vi "Aplicatie_trigger.vi"() -> ()   [LabVIEW 2020]
uses:
  994e1307-8dd3-4d9d-b32b-35e3dfa9da5e.vi
  <instrlib>/Agilent 34401/Agilent 34401.lvlib
  \\bucgroup.buc.infineon.com\sc/Internship/CV/2023/Tektronix DPO MSO 2000 4000 Series/Tektronix DPO MSO 2000 4000 Series.lvlib
panel:
  out "error out 2":errorcluster
  out "error out 4":errorcluster
  out "VISA Refnum out":refnum<visa-resource-name>
  in  "Press for measurement":bool
  in  "error in (no error)":errorcluster
  in  "stop":bool
  in  "Select index of measurement:":string(combo)
  in  "Select channel":string(combo)
  in  "Select state:":string(combo)
  in  "Select measurement":string(combo)
  in  "Select statistics's state:":string(combo)
  in  "Select type of histogram:":string(combo)
  in  "Select channel for histogram:":string(combo)
  in  "Select second  transition:":string(combo)
  in  "Select first transition:":string(combo)
  in  "Select polarity:":string(combo)
  in  "Select second channel:":string(combo)
  in  "Select first channel:":string(combo)
  in  "Press for Delta[ms]":bool
  out "Delta[ms]":string
  in  "Cursors Waveform":string(combo)
  in  "SELECT STATE":string(combo)
  in  "SELECT CHANNEL FOR STATE":string(combo)
  in  "Position":dbl
  in  "Select Horizontal position's state:":string(combo)
  in  "Horizontal":dbl step=1.6e-07
  in  "Horizontal Scale":string(combo)
  in  "SELECT CHANNEL FOR SCALE":string(combo)
  in  "Vertical Scale":dbl
  in  "Linked":string(combo)
  in  "Press for Settings for the horizontal bar cursors":bool
  out "Settings for horizontal bar cursors":string
  in  "Press for Settings for the vertical bar cursors":bool
  out "Settings for VERTICAL bar cursors":string
  in  "Select the units":string(combo)
  in  "Press for Delta[mV]":bool
  out "Delta[mV]":string
  in  "Horizontal Cursor 2":dbl(slide) step=0.01 scale=-10.0..10.0
  in  "Horizontal Cursor 1":dbl(slide) step=0.01 scale=-10.0..10.0
  in  "Vertical Cursor 2":dbl(slide) scale=-2e-05..2e-05
  in  "Vertical Cursor 1":dbl(slide) step=0.01 scale=-2e-05..2e-05
  in  "Dots Only":string(combo)
  in  "Select Record Length":string(combo)
  in  "Select mode":string(combo)
  in  "Select bandwidth:":string(combo)
  in  "Select termination:":string(combo)
  in  "Select invert:":string(combo)
  in  "Select coupling:":string(combo)
  in  "Select channel:":string(combo)
  in  "VISA resource name":refnum<visa-resource-name>="USB0::0x0699::0x0401::C000915::INSTR"
  out "error out":errorcluster
  in  "Delay 2":dbl
  in  "Trig OUT 2":string(combo)
  in  "Burst state 2":string(combo)
  in  "Trigger Setup 2":string(combo)
  in  "Number of cycles 2":dbl
  in  "Edge Time 2":dbl
  in  "Pulse Width 2":dbl
  in  "HighLevel 2":dbl
  in  "LowLevel 2":dbl
  in  "Amplitude 2":dbl
  in  "Select function":string(combo)
  in  "Period 2":dbl
  in  "Delay":dbl
  in  "Trig OUT":string(combo)
  in  "Burst state":string(combo)
  in  "Trigger Setup":string(combo)
  in  "Number of cycles":dbl
  in  "Edge Time":dbl
  in  "Pulse Width":dbl
  in  "HighLevel":dbl
  in  "LowLevel":dbl
  in  "Amplitude":dbl
  in  "Select function":string(combo)
  in  "Period":dbl
  # "Configure left waveform generator"
  # "Configure right waveform generator"
  # "Trigger Error"
  # "Measure"
  # "Channel Config"
  # "Acquire"
  # "Add measurement:"
  # "Configure Delay:"
  # "Statistics's state:"
  # "Waveform Histograms:"
  # "Cursors"
  # "Vertical  position"
  # "Vertical scale"
  # "Channel Management"
  # "Horizontal scale"
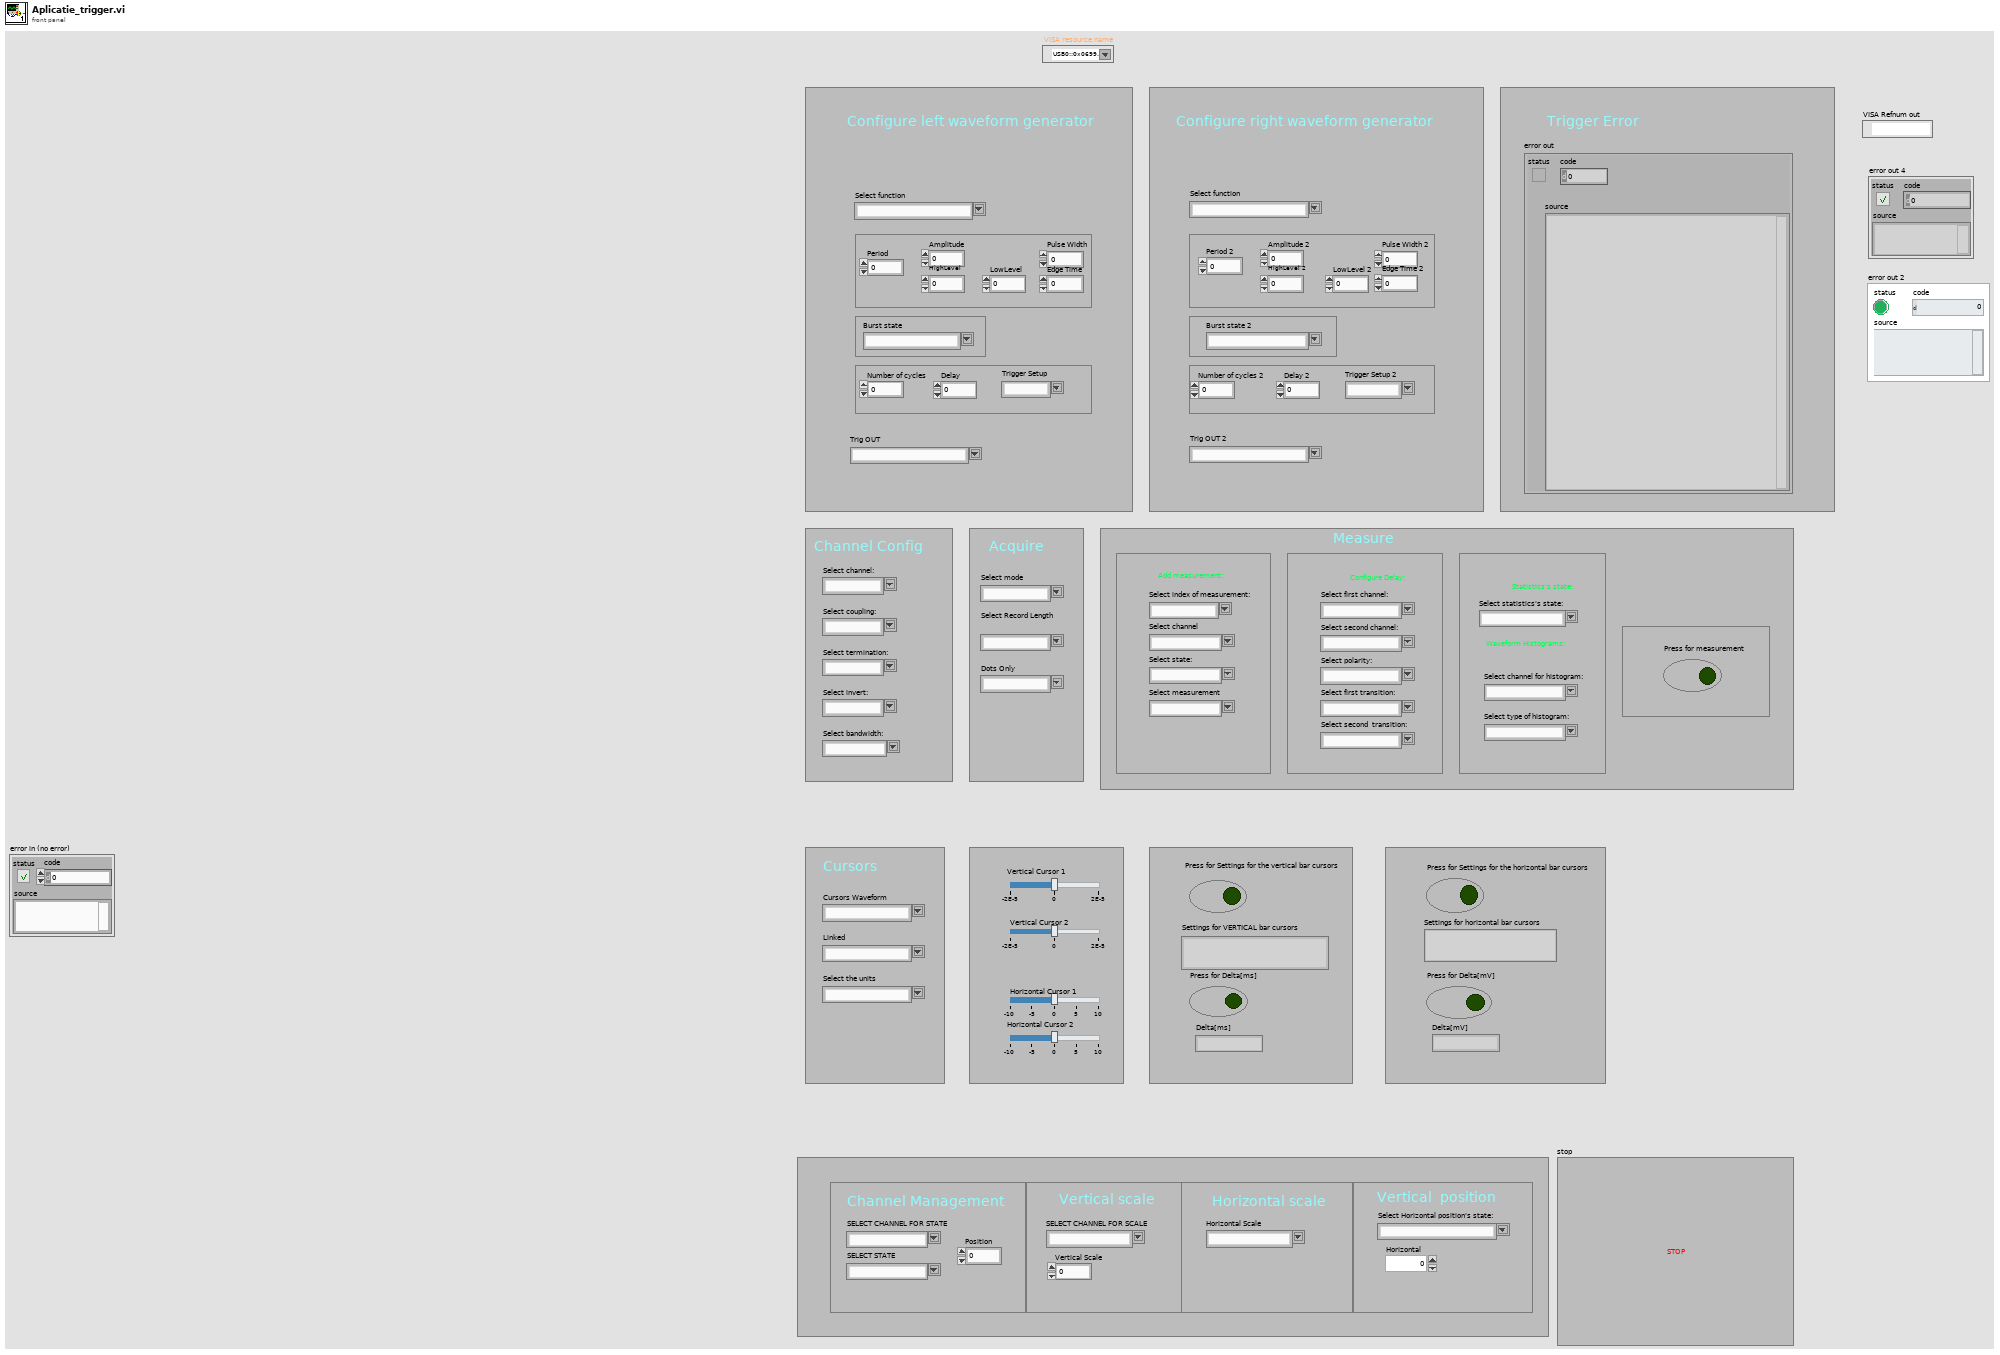
[diagram p1: front panel]
types:
  T1 = enum16{"open", "open or create", "create or replace", "create", "open (read-only)"}
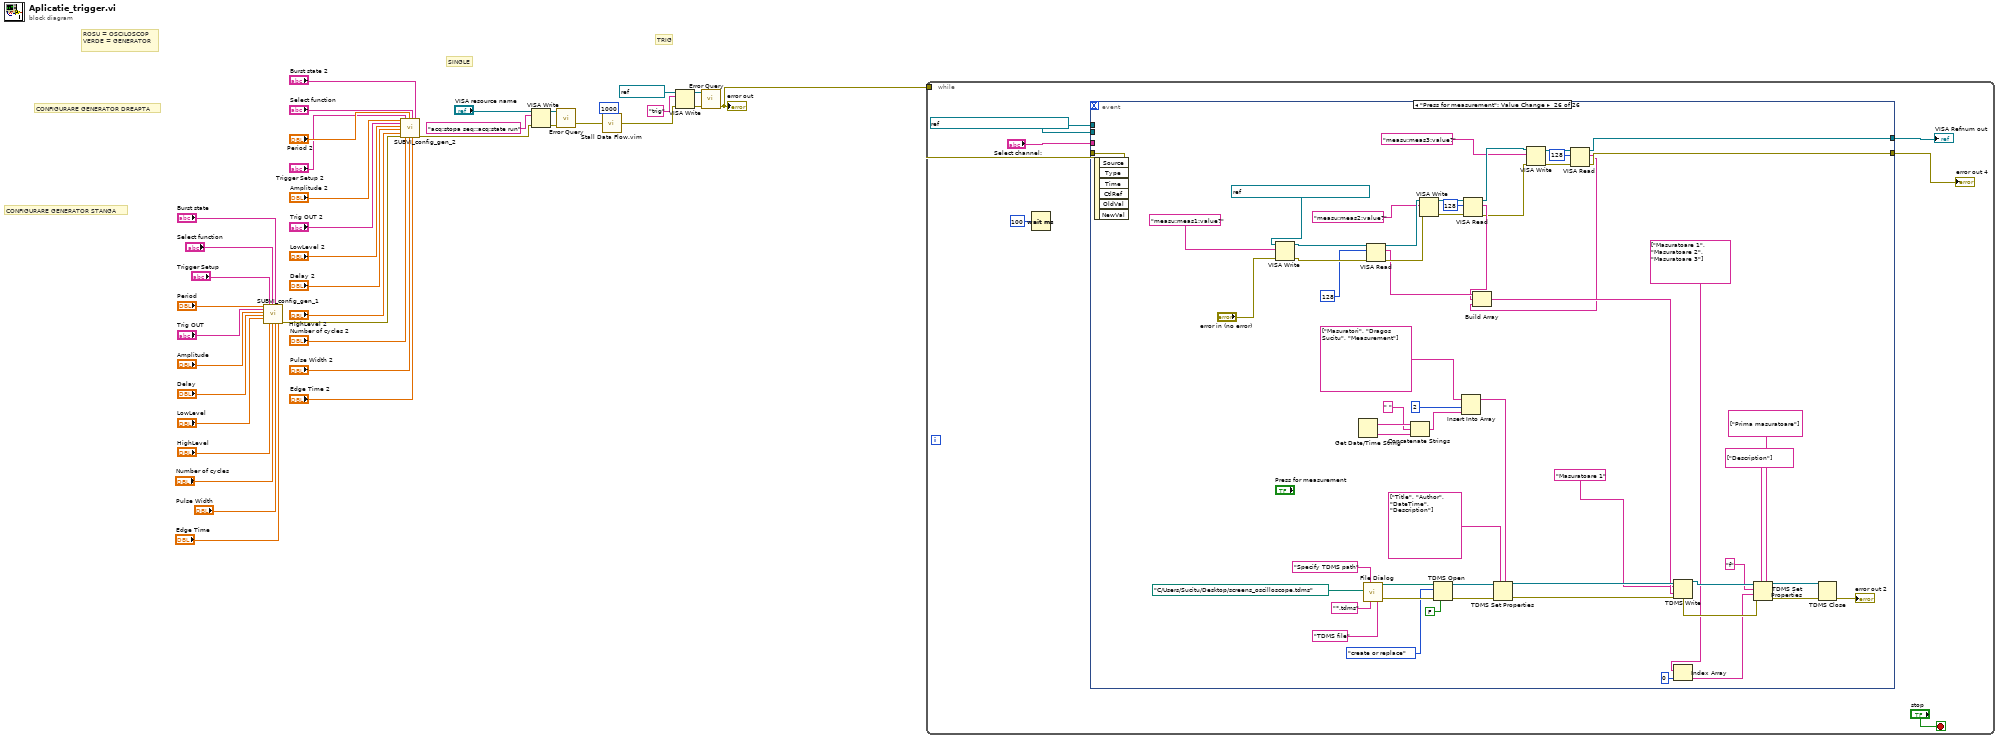
[diagram p0: block diagram]
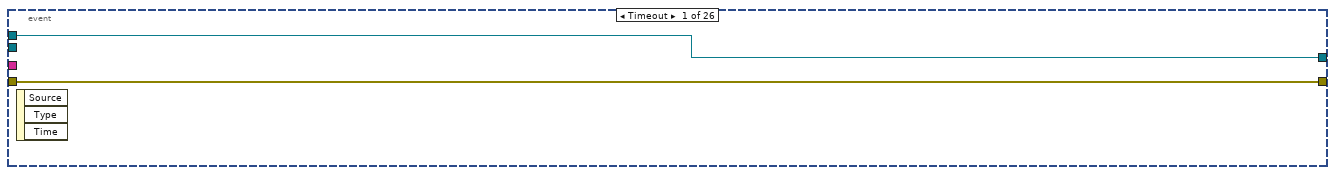
[diagram p2: hidden frame]
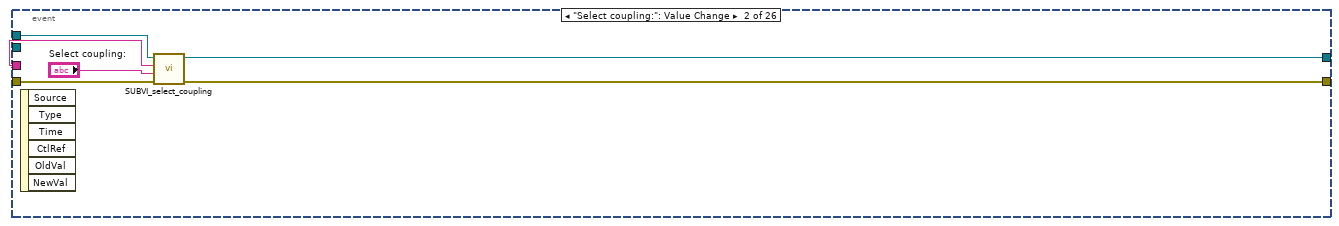
[diagram p3: hidden frame]
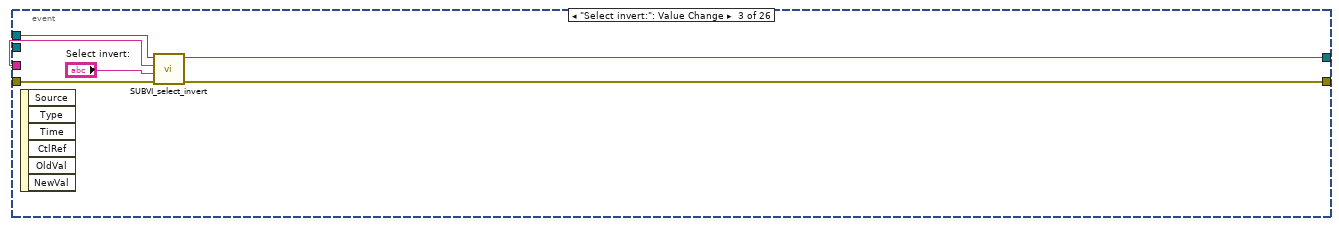
[diagram p4: hidden frame]
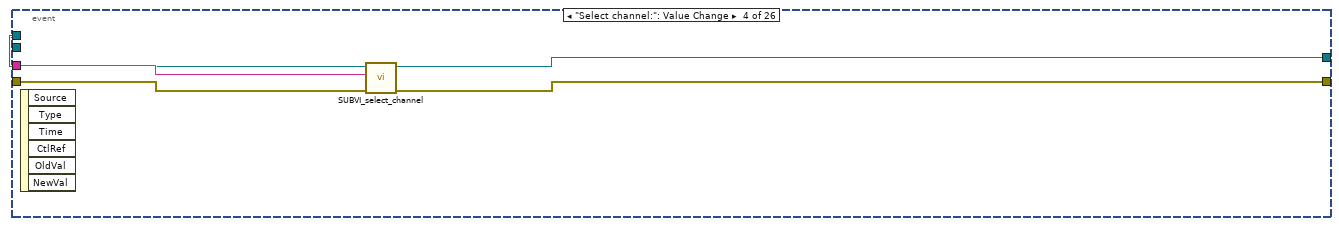
[diagram p5: hidden frame]
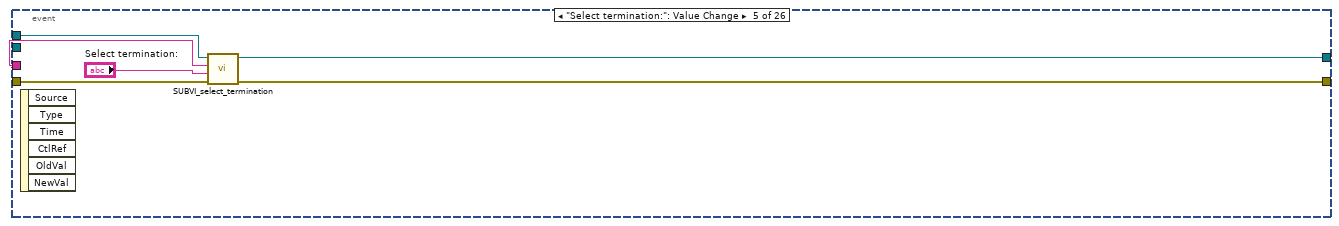
[diagram p6: hidden frame]
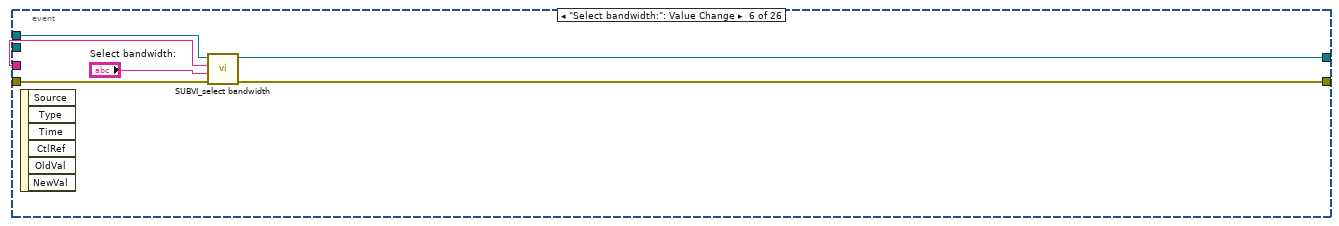
[diagram p7: hidden frame]
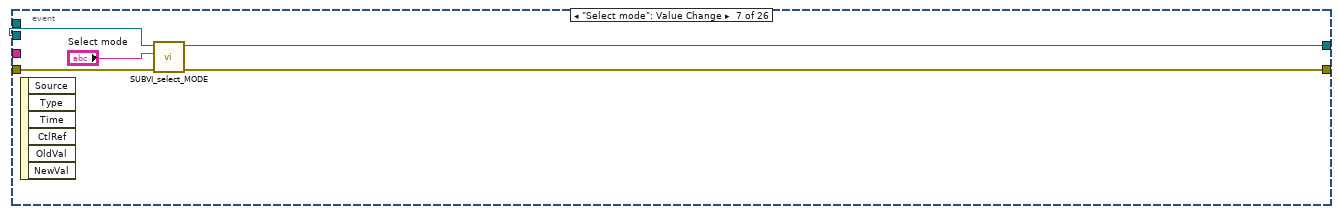
[diagram p8: hidden frame]
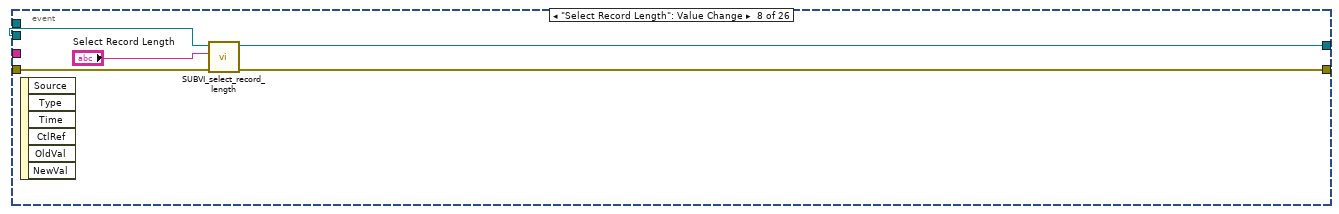
[diagram p9: hidden frame]
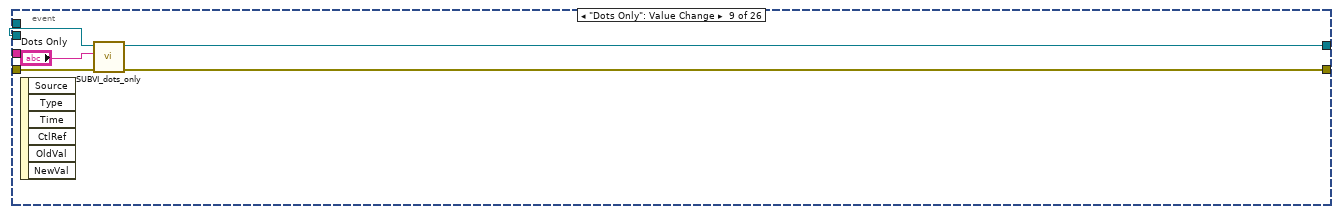
[diagram p10: hidden frame]
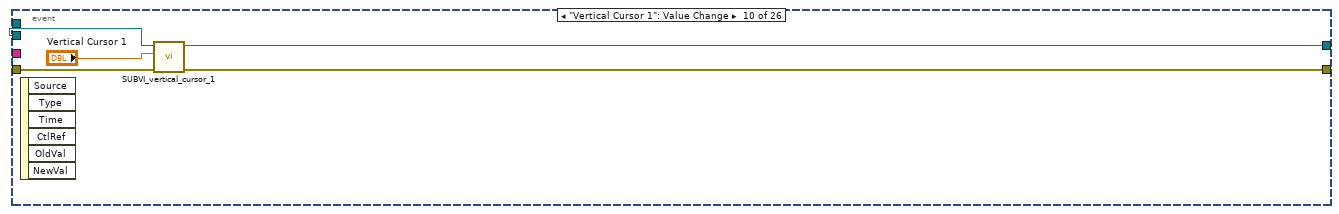
[diagram p11: hidden frame]
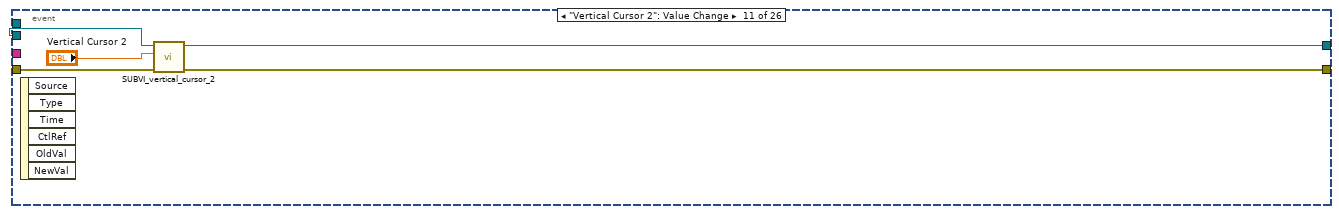
[diagram p12: hidden frame]
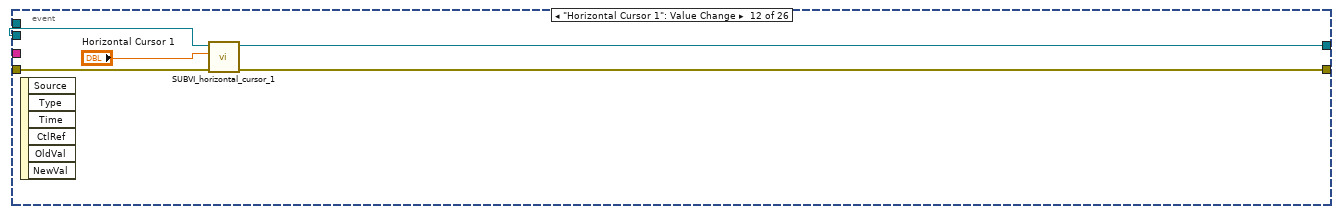
[diagram p13: hidden frame]
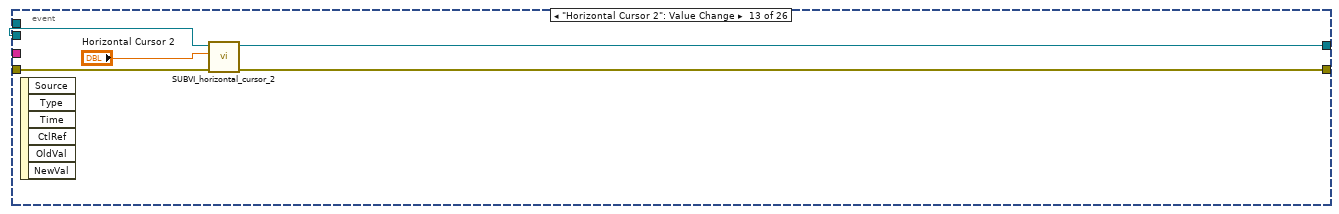
[diagram p14: hidden frame]
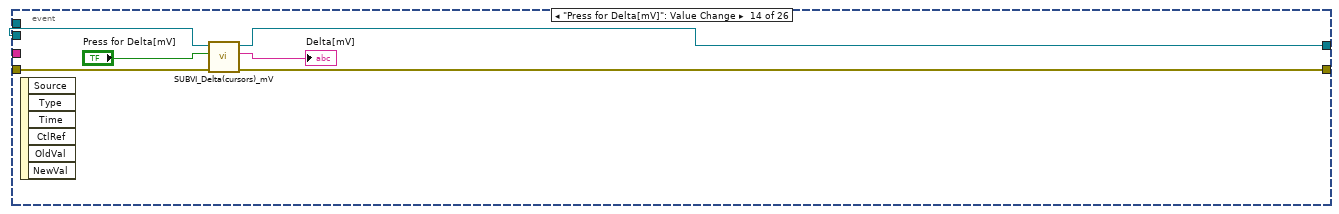
[diagram p15: hidden frame]
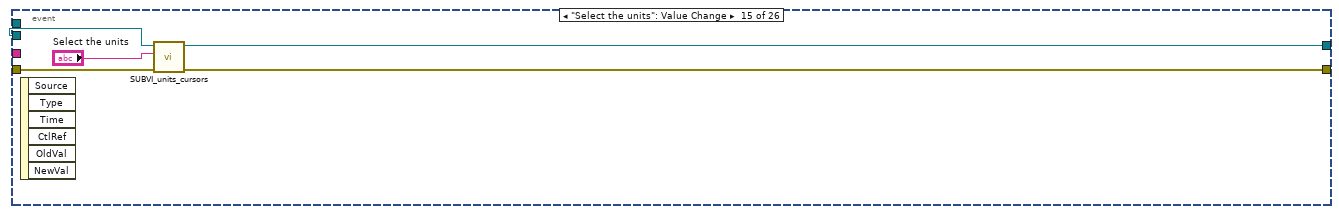
[diagram p16: hidden frame]
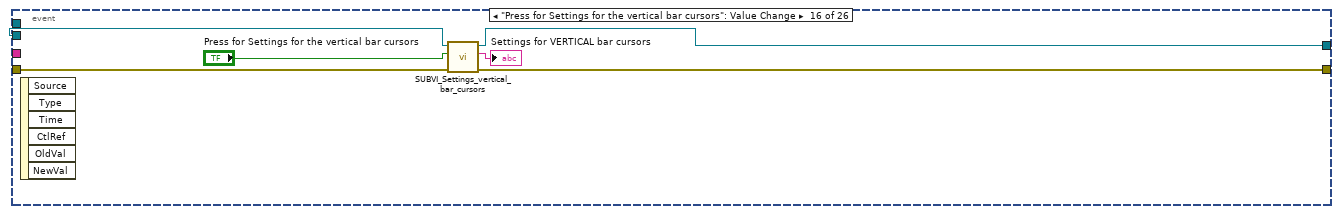
[diagram p17: hidden frame]
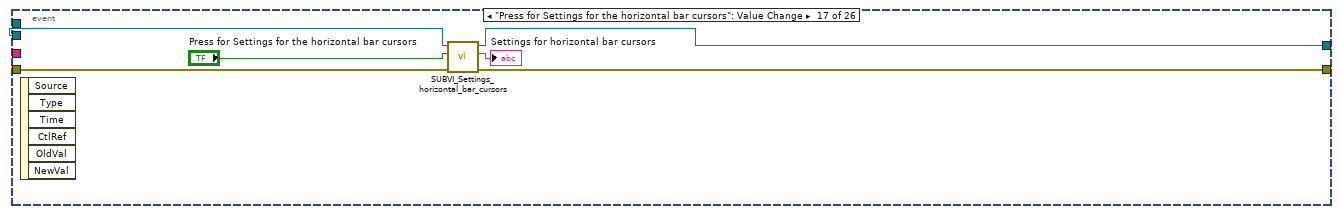
[diagram p18: hidden frame]
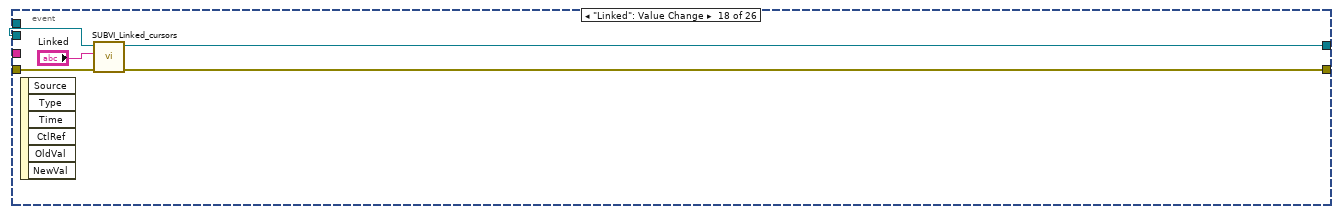
[diagram p19: hidden frame]
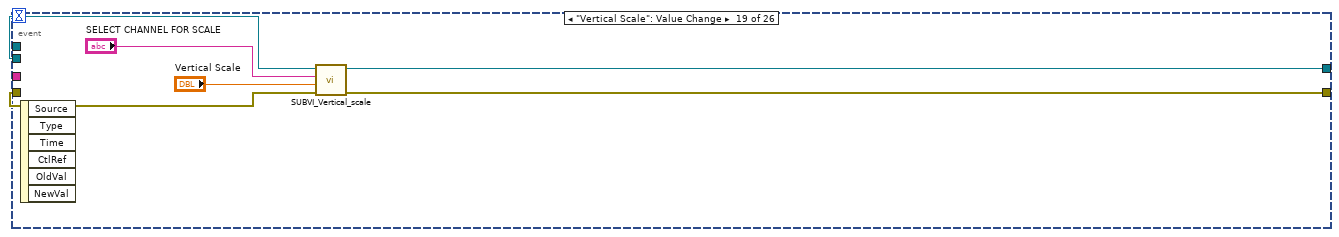
[diagram p20: hidden frame]
diagram:
  # "SINGLE"
  # "TRIG"
  # "CONFIGURARE GENERATOR DREAPTA"
  # "CONFIGURARE GENERATOR STANGA"
  # "ROSU = OSCILOSCOP\nVERDE = GENERATOR"
  n1 = call "SUBVI_config_gen_1.vi"("Period"="Period", "Trig OUT"="Trig OUT", "Amplitude"="Amplitude", "Delay"="Delay", "LowLevel"="LowLevel", "Trigger Setup"="Trigger Setup", "HighLevel"="HighLevel", "Select function"="Select function", "Number of cycles"="Number of cycles", "Burst state"="Burst state", "Pulse Width"="Pulse Width", "Edge Time"="Edge Time") -> ("error out"=w38:errorcluster)  [unwired: 7 in]
  n2 = call "SUBVI_config_gen_2.vi"("Amplitude in"="Amplitude 2", "Trig OUT in"="Trig OUT 2", "LowLevel in"="LowLevel 2", "Delay in"="Delay 2", "HighLevel in"="HighLevel 2", "error in (no error)"=w38, "Trigger Setup in"="Trigger Setup 2", "Number of cycles in"="Number of cycles 2", "Period in"="Period 2", "Pulse Width in"="Pulse Width 2", "Select function"="Select function", "Edge Time in"="Edge Time 2", "Burst state in"="Burst state 2") -> ("error out"=w37:errorcluster)  [unwired: 6 in]
  n3 = VISA Write(VISA resource name="VISA resource name", write buffer="acq:stopa seq;:acq:state run", error in (no error)=w37) -> (VISA resource name out=w10:refnum<visa-resource-name>, error out=w12:errorcluster)  [unwired: 1 out]
  n4 = call <instrlib>:"Error Query.vi"("error in (no error)"=w12, "VISA resource name"=w10) -> ("error out"=w2:errorcluster)  [unwired: 6 in, 3 out]
  n5 = call "Stall Data Flow.vim"("value in"=w2, "milliseconds to wait"=u32 1000) -> ("value out"=w1:errorcluster)  [unwired: 1 out]
  n6 = VISA Write(VISA resource name=refnum<visa-resource-name> "STANGA", write buffer="trig", error in (no error)=w1) -> (VISA resource name out=w8:refnum<visa-resource-name>, error out=w7:errorcluster)  [unwired: 1 out]
  n7 = call <instrlib>:"Error Query.vi"("error in (no error)"=w7, "VISA resource name"=w8) -> ("error out"=w4:errorcluster)  [unwired: 6 in, 3 out]
  "error out" <- w4
  n8 = while {
    tunnel: w4 -> [w43]
    stop <- "stop" stop-if-true
    w41 = refnum<visa-resource-name> "USB0::0x0699::0x0401::C000915::INSTR" ("VISA resource name")
    n9 = Wait (ms)(milliseconds to wait=u32 100) -> ()  [unwired: 1 out]
    n10 = event shown="[25] \"Press for measurement\": Value Change" {
      selector: _ -> [_ _ _ _ _ _ _ _ _ _ _ _ _ _ _ _ _ _ _ _ _ _ _ _ _ _]
      dyn-events: _ -> [_ _ _ _ _ _ _ _ _ _ _ _ _ _ _ _ _ _ _ _ _ _ _ _ _ _]
      timeout: _ -> [_ _ _ _ _ _ _ _ _ _ _ _ _ _ _ _ _ _ _ _ _ _ _ _ _ _]
      tunnel: w43 -> [w47 w52 w57 w62 w66 w72 w80 w85 w89 w94 w99 w104 w109 w115 w120 w126 w132 w137 w142 w148 w153 w159 w166 w172 w183 _]
      tunnel: "Select channel:" -> [_ w49 w59 w64 w70 w76 _ _ _ _ _ _ _ _ _ _ _ _ _ _ _ _ _ _ _ _]
      tunnel: w41 -> [w46 w48 w54 w63 w65 w71 _ _ _ _ _ _ _ _ _ _ _ _ _ _ _ _ _ _ _ _]
      tunnel: w41 -> [_ _ _ _ _ _ w77 w82 w90 w95 w100 w105 w110 w116 w121 w127 w133 w138 w143 w149 w154 w160 w167 w173 w182 _]
      tunnel: [w46 w51 w56 w60 w68 w74 w79 w84 w88 w93 w98 w103 w108 w114 w119 w125 w131 w136 w141 w147 w152 w158 w165 w171 w176 w194] -> w40
      tunnel: [w47 w50 w55 w61 w67 w73 w78 w83 w87 w92 w97 w102 w107 w113 w118 w124 w130 w135 w140 w146 w151 w157 w164 w170 w175 w193] -> w39
      event Timeout {
        n11 = event-data() -> ()  [unwired: 1 in, 3 out]
      }
      event "Select coupling:": Value Change {
        n12 = event-data() -> ()  [unwired: 1 in, 6 out]
        n13 = call "SUBVI_select_coupling.vi"("error in (no error)"=w52, "Select coupling:"="Select coupling:", "Select channel:"=w49, "VISA Refnum in"=w48) -> ("error out"=w50:errorcluster, "VISA Refnum out"=w51:refnum<visa-resource-name>)  [unwired: 6 in]
      }
      event "Select invert:": Value Change {
        n14 = event-data() -> ()  [unwired: 1 in, 6 out]
        n15 = call "SUBVI_select_invert.vi"("error in (no error)"=w57, "Select invert:"="Select invert:", "Select channel:"=w59, "VISA Refnum in"=w54) -> ("error out"=w55:errorcluster, "VISA Refnum out"=w56:refnum<visa-resource-name>)  [unwired: 6 in]
      }
      event "Select channel:": Value Change {
        n16 = event-data() -> ()  [unwired: 1 in, 6 out]
        n17 = call "SUBVI_select_channel.vi"("error in (no error)"=w62, "Select channel:"=w64, "VISA Refnum in"=w63) -> ("error out"=w61:errorcluster, "VISA Refnum out"=w60:refnum<visa-resource-name>)  [unwired: 7 in]
      }
      event "Select termination:": Value Change {
        n18 = event-data() -> ()  [unwired: 1 in, 6 out]
        n19 = call "SUBVI_select_termination.vi"("error in (no error)"=w66, "Select termination:"="Select termination:", "Select channel:"=w70, "VISA Refnum in"=w65) -> ("error out"=w67:errorcluster, "VISA Refnum out"=w68:refnum<visa-resource-name>)  [unwired: 6 in]
      }
      event "Select bandwidth:": Value Change {
        n20 = event-data() -> ()  [unwired: 1 in, 6 out]
        n21 = call "SUBVI_select bandwidth.vi"("error in (no error)"=w72, "Select bandwidth:"="Select bandwidth:", "Select channel:"=w76, "VISA Refnum in"=w71) -> ("error out"=w73:errorcluster, "VISA Refnum out"=w74:refnum<visa-resource-name>)  [unwired: 6 in]
      }
      event "Select mode": Value Change {
        n22 = event-data() -> ()  [unwired: 1 in, 6 out]
        n23 = call "SUBVI_select_MODE.vi"("error in (no error)"=w80, "Select mode"="Select mode", "VISA Refnum in"=w77) -> ("error out"=w78:errorcluster, "VISA Refnum out"=w79:refnum<visa-resource-name>)  [unwired: 7 in]
      }
      event "Select Record Length": Value Change {
        n24 = event-data() -> ()  [unwired: 1 in, 6 out]
        n25 = call "SUBVI_select_record_length.vi"("error in (no error)"=w85, "Select Record Length"="Select Record Length", "VISA Refnum in"=w82) -> ("error out"=w83:errorcluster, "VISA Refnum out"=w84:refnum<visa-resource-name>)  [unwired: 7 in]
      }
      event "Dots Only": Value Change {
        n26 = event-data() -> ()  [unwired: 1 in, 6 out]
        n27 = call "SUBVI_dots_only.vi"("error in (no error)"=w89, "Dots Only"="Dots Only", "VISA Refnum in"=w90) -> ("error out"=w87:errorcluster, "VISA Refnum out"=w88:refnum<visa-resource-name>)  [unwired: 7 in]
      }
      event "Vertical Cursor 1": Value Change {
        n28 = event-data() -> ()  [unwired: 1 in, 6 out]
        n29 = call "SUBVI_vertical_cursor_1.vi"("error in (no error)"=w94, "Vertical Cursor 1"="Vertical Cursor 1", "VISA Refnum in"=w95) -> ("error out"=w92:errorcluster, "VISA Refnum out"=w93:refnum<visa-resource-name>)  [unwired: 7 in]
      }
      event "Vertical Cursor 2": Value Change {
        n30 = event-data() -> ()  [unwired: 1 in, 6 out]
        n31 = call "SUBVI_vertical_cursor_2.vi"("error in (no error)"=w99, "Vertical Cursor in"="Vertical Cursor 2", "VISA Refnum in"=w100) -> ("error out"=w97:errorcluster, "VISA Refnum out"=w98:refnum<visa-resource-name>)  [unwired: 7 in]
      }
      event "Horizontal Cursor 1": Value Change {
        n32 = event-data() -> ()  [unwired: 1 in, 6 out]
        n33 = call "SUBVI_horizontal_cursor_1.vi"("error in (no error)"=w104, "Horizontal Cursor 1"="Horizontal Cursor 1", "VISA Refnum in"=w105) -> ("error out"=w102:errorcluster, "VISA Refnum out"=w103:refnum<visa-resource-name>)  [unwired: 7 in]
      }
      event "Horizontal Cursor 2": Value Change {
        n34 = event-data() -> ()  [unwired: 1 in, 6 out]
        n35 = call "SUBVI_horizontal_cursor_2.vi"("error in (no error)"=w109, "Horizontal Cursor in"="Horizontal Cursor 2", "VISA Refnum in"=w110) -> ("error out"=w107:errorcluster, "VISA Refnum out"=w108:refnum<visa-resource-name>)  [unwired: 7 in]
      }
      event "Press for Delta[mV]": Value Change {
        n36 = event-data() -> ()  [unwired: 1 in, 6 out]
        n37 = call "SUBVI_Delta(cursors)_mV.vi"("error in (no error)"=w115, "Press for Delta[mV]"="Press for Delta[mV]", "VISA Refnum in"=w116) -> ("error out"=w113:errorcluster, "Delta[mV]"=→"Delta[mV]":string, "VISA Refnum out"=w114:refnum<visa-resource-name>)  [unwired: 6 in]
      }
      event "Select the units": Value Change {
        n38 = event-data() -> ()  [unwired: 1 in, 6 out]
        n39 = call "SUBVI_units_cursors.vi"("error in (no error)"=w120, "Select the units"="Select the units", "VISA Refnum in"=w121) -> ("error out"=w118:errorcluster, "VISA Refnum out"=w119:refnum<visa-resource-name>)  [unwired: 7 in]
      }
      event "Press for Settings for the vertical bar cursors": Value Change {
        n40 = event-data() -> ()  [unwired: 1 in, 6 out]
        n41 = call "SUBVI_Settings_vertical_bar_cursors.vi"("error in (no error)"=w126, "Press for Settings for the vertical bar cursors"="Press for Settings for the vertical bar cursors", "VISA Refnum in"=w127) -> ("error out"=w124:errorcluster, "Settings for horizontal bar cursors"=→"Settings for VERTICAL bar cursors":string, "VISA Refnum out"=w125:refnum<visa-resource-name>)  [unwired: 6 in]
      }
      event "Press for Settings for the horizontal bar cursors": Value Change {
        n42 = event-data() -> ()  [unwired: 1 in, 6 out]
        n43 = call "SUBVI_Settings_horizontal_bar_cursors.vi"("error in (no error)"=w132, "Press for Settings for the horizontal bar cursors"="Press for Settings for the horizontal bar cursors", "VISA Refnum in"=w133) -> ("error out"=w130:errorcluster, "Settings for horizontal bar cursors 2"=→"Settings for horizontal bar cursors":string, "VISA Refnum out"=w131:refnum<visa-resource-name>)  [unwired: 6 in]
      }
      event "Linked": Value Change {
        n44 = event-data() -> ()  [unwired: 1 in, 6 out]
        n45 = call "SUBVI_Linked_cursors.vi"("error in (no error)"=w137, "Linked"="Linked", "VISA Refnum in"=w138) -> ("error out"=w135:errorcluster, "VISA Refnum out"=w136:refnum<visa-resource-name>)  [unwired: 7 in]
      }
      event "Vertical Scale": Value Change {
        n46 = event-data() -> ()  [unwired: 1 in, 6 out]
        n47 = call "SUBVI_Vertical_scale.vi"("error in (no error)"=w142, "Vertical Scale"="Vertical Scale", "SELECT CHANNEL FOR SCALE"="SELECT CHANNEL FOR SCALE", "VISA Refnum in"=w143) -> ("error out"=w140:errorcluster, "VISA Refnum out"=w141:refnum<visa-resource-name>)  [unwired: 6 in]
      }
      event "Horizontal Scale": Value Change {
        n48 = event-data() -> ()  [unwired: 1 in, 6 out]
        n49 = call "SUBVI_Horizontal_scale.vi"("error in (no error)"=w148, "Horizontal Scale"="Horizontal Scale", "VISA Refnum in"=w149) -> ("error out"=w146:errorcluster, "VISA Refnum out"=w147:refnum<visa-resource-name>)  [unwired: 7 in]
      }
      event "Horizontal": Value Change {
        n50 = event-data() -> ()  [unwired: 1 in, 6 out]
        n51 = call "SUBVI_Horizontal_position.vi"("error in (no error)"=w153, "Select Horizontal position's state:"="Select Horizontal position's state:", "Horizontal"="Horizontal", "VISA Refnum in"=w154) -> ("error out"=w151:errorcluster, "VISA Refnum out"=w152:refnum<visa-resource-name>)  [unwired: 6 in]
      }
      event "SELECT CHANNEL FOR STATE", "Position": Value Change {
        n52 = event-data() -> ()  [unwired: 1 in, 6 out]
        n53 = call "SUBVI_Select_channel_for_state.vi"("SELECT STATE"="SELECT STATE", "error in (no error)"=w159, "Position"="Position", "SELECT CHANNEL FOR STATE"="SELECT CHANNEL FOR STATE", "VISA Refnum in"=w160) -> ("error out"=w157:errorcluster, "VISA Refnum out"=w158:refnum<visa-resource-name>)  [unwired: 5 in]
      }
      event "Cursors Waveform": Value Change {
        n54 = event-data() -> ()  [unwired: 1 in, 6 out]
        n55 = call "SUBVI_Cursors_waveform.vi"("error in (no error)"=w166, "Cursors Waveform"="Cursors Waveform", "VISA Refnum in"=w167) -> ("error out"=w164:errorcluster, "VISA Refnum out"=w165:refnum<visa-resource-name>)  [unwired: 7 in]
      }
      event "Press for Delta[ms]": Value Change {
        n56 = event-data() -> ()  [unwired: 1 in, 6 out]
        n57 = call "SUBVI_Delta(cursors)_ms.vi"("error in (no error)"=w172, "Press for Delta[ms]"="Press for Delta[ms]", "VISA Refnum in"=w173) -> ("error out"=w170:errorcluster, "Delta[ms]"=→"Delta[ms]":string, "VISA Refnum out"=w171:refnum<visa-resource-name>)  [unwired: 6 in]
      }
      event "Select channel", "Select state:", "Select measurement", "Select second  transition:", "Select first transition:", "Select polarity:", "Select second channel:", "Select first channel:", "Select statistics's state:", "Select type of histogram:", "Select channel for histogram:": Value Change {
        n58 = event-data() -> ()  [unwired: 1 in, 6 out]
        n59 = call "SUBVI_add_measurement.vi"("VISA Refnum in"=w182, "Select index of measurement:"="Select index of measurement:", "Select channel for histogram:"="Select channel for histogram:", "Select measurement"="Select measurement", "Select type of histogram:"="Select type of histogram:", "error in (no error)"=w183, "Select channel"="Select channel", "Select state:"="Select state:", "Select second channel:"="Select second channel:", "Select polarity:"="Select polarity:", "Select first channel:"="Select first channel:", "Select first transition:"="Select first transition:", "Select statistics's state:"="Select statistics's state:", "Select second  transition:"="Select second  transition:") -> ("VISA Refnum out"=w176:refnum<visa-resource-name>, "error out"=w175:errorcluster)  [unwired: 4 in]
      }
      event "Press for measurement": Value Change {
        n60 = event-data() -> ()  [unwired: 1 in, 6 out]
        n61 = VISA Write(VISA resource name=refnum<visa-resource-name> "USB0::0x0699::0x0401::C000915::INSTR", write buffer="measu:meas1:value?", error in (no error)="error in (no error)") -> (VISA resource name out=w245:refnum<visa-resource-name>, error out=w246:errorcluster)  [unwired: 1 out]
        n62 = Get Date/Time String() -> (date string=w225:string, time string=w223:string)  [unwired: 3 in]
        n63 = call "File Dialog"("start path"=path "C:/Users/Sucitu/Desktop/screens_oscilloscope.tdms", "prompt"="Specify TDMS path", "pattern (all files)"="*.tdms", "pattern label"="TDMS file") -> ("selected path"=w237:path, "error out"=w236:errorcluster)  [unwired: 8 in, 2 out]
        n64 = VISA Read(VISA resource name=w245, byte count=u32 128, error in (no error)=w246) -> (VISA resource name out=w210:refnum<visa-resource-name>, read buffer=w205:string, error out=w209:errorcluster)  [unwired: 1 out]
        n65 = Concatenate Strings(w225, " " ("string"), w223) -> (w224:string)
        n66 = VISA Write(VISA resource name=w210, write buffer="measu:meas2:value?", error in (no error)=w209) -> (VISA resource name out=w208:refnum<visa-resource-name>, error out=w207:errorcluster)  [unwired: 1 out]
        n67 = TDMS Open(6:FALSE ("disable buffering? (T)"), 8:w236, 10:T1."create or replace" ("operation (0:open)"), 11:w237) -> (0:w230:errorcluster, 3:w231:refnum<k34>)  [unwired: 3 in]
        n68 = Insert Into Array(array=string[] ["Masuratori", "Dragos Sucitu", "Measurement"] ("property names"), index=2, new element=w224) -> (w227:string[])
        n69 = VISA Read(VISA resource name=w208, byte count=u32 128, error in (no error)=w207) -> (VISA resource name out=w195:refnum<visa-resource-name>, read buffer=w204:string, error out=w196:errorcluster)  [unwired: 1 out]
        n70 = TDMS Set Properties(5:w227, 7:string[] ["Title", "Author", "DateTime", "Description"] ("property names"), 8:w230, 11:w231) -> (0:w216:errorcluster, 3:w217:refnum<k34>)  [unwired: 2 in, 2 out]
        n71 = VISA Write(VISA resource name=w195, write buffer="measu:meas3:value?", error in (no error)=w196) -> (VISA resource name out=w199:refnum<visa-resource-name>, error out=w198:errorcluster)  [unwired: 1 out]
        n72 = VISA Read(VISA resource name=w199, byte count=u32 128, error in (no error)=w198) -> (VISA resource name out=w194:refnum<visa-resource-name>, read buffer=w191:string, error out=w193:errorcluster)  [unwired: 1 out]
        n73 = Build Array(w205, w204, w191) -> (w203:string[])
        n74 = TDMS Write(0:w217, 5:"Masuratoare 1" ("channel name(s) in (Untitled)"), 9:w203, 11:w216) -> (4:w214:refnum<k34>, 15:w215:errorcluster)  [unwired: 2 in, 2 out]
        n75 = Index Array(array=string[] ["Masuratoare 1", "Masuratoare 2", "Masuratoare 3"] ("property names"), index=0) -> (element=w212:string)
        n76 = TDMS Set Properties(5:string[] ["Prima masuratoare"] ("property names"), 7:string[] ["Description"] ("property names"), 8:w215, 9:w212, 10:"f" ("group name"), 11:w214) -> (0:w218:errorcluster, 3:w219:refnum<k34>)  [unwired: 2 out]
        n77 = TDMS Close(8:w218, 11:w219) -> (0:→"error out 2":errorcluster)  [unwired: 1 out]
      }
    }
    "VISA Refnum out" <- w40
    "error out 4" <- w39
  }
